vi "capacimetro_adv.vi"() -> ()   [LabVIEW 2019]
uses:
  <vilib>/Analysis/1siggen.llb/Ramp Pattern by Samples.vi
  <vilib>/Instr/_visa.llb/VISA Configure Serial Port (Instr).vi
  <vilib>/Analysis/NI_AALBase.lvlib
  <vilib>/Analysis/NI_AALPro.lvlib
panel:
  out "tau":dbl
  in  "Medie":bool
  out "ADC NL":cluster{dbl[], dbl[]}(graph)
  out "Residui":cluster{dbl[], dbl[]}(graph)
  out "Segnale":cluster{dbl[], "Best Exponential Fit":dbl[]}[](graph)
  out "C[pF]":dbl
  in  "Rs[kohm]":dbl
  out "offset":dbl
  in  "dT":i32
  in  "begin":i32
  in  "length":i32
  in  "stop":bool
  in  "VISA resource name":refnum<visa-resource-name>
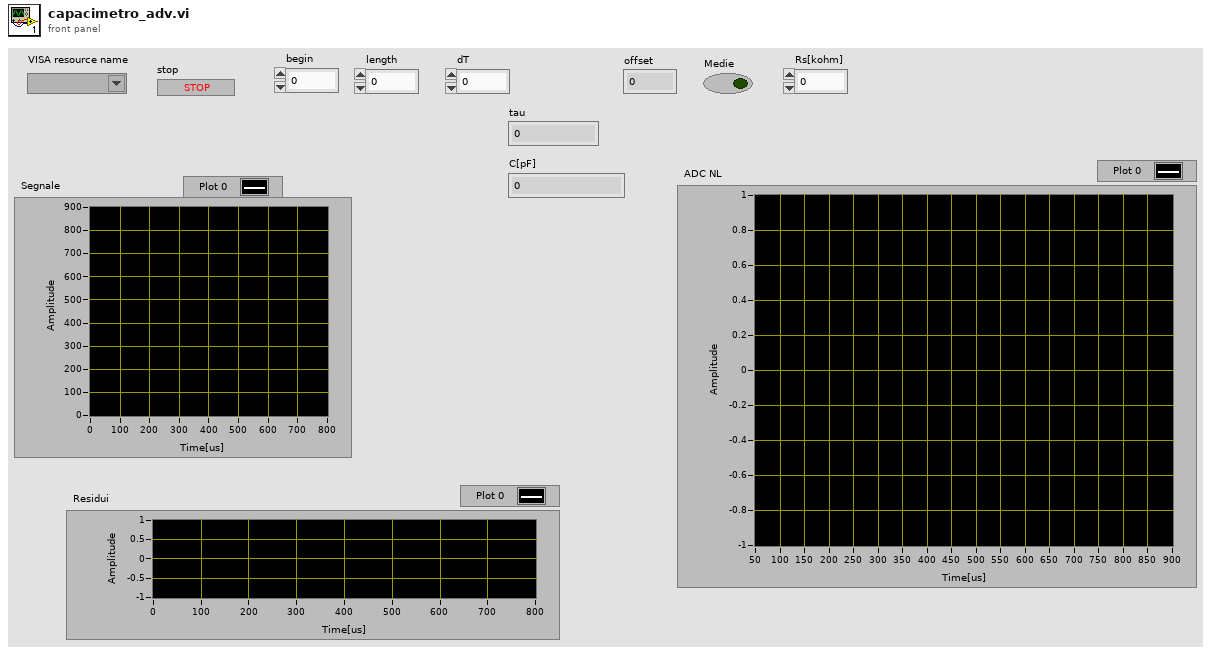
[diagram p1: front panel]
types:
  T1 = cluster{"amp min":dbl, "amp max":dbl, "damping min":dbl, "damping max":dbl, "offset min":dbl, "offset max":dbl}
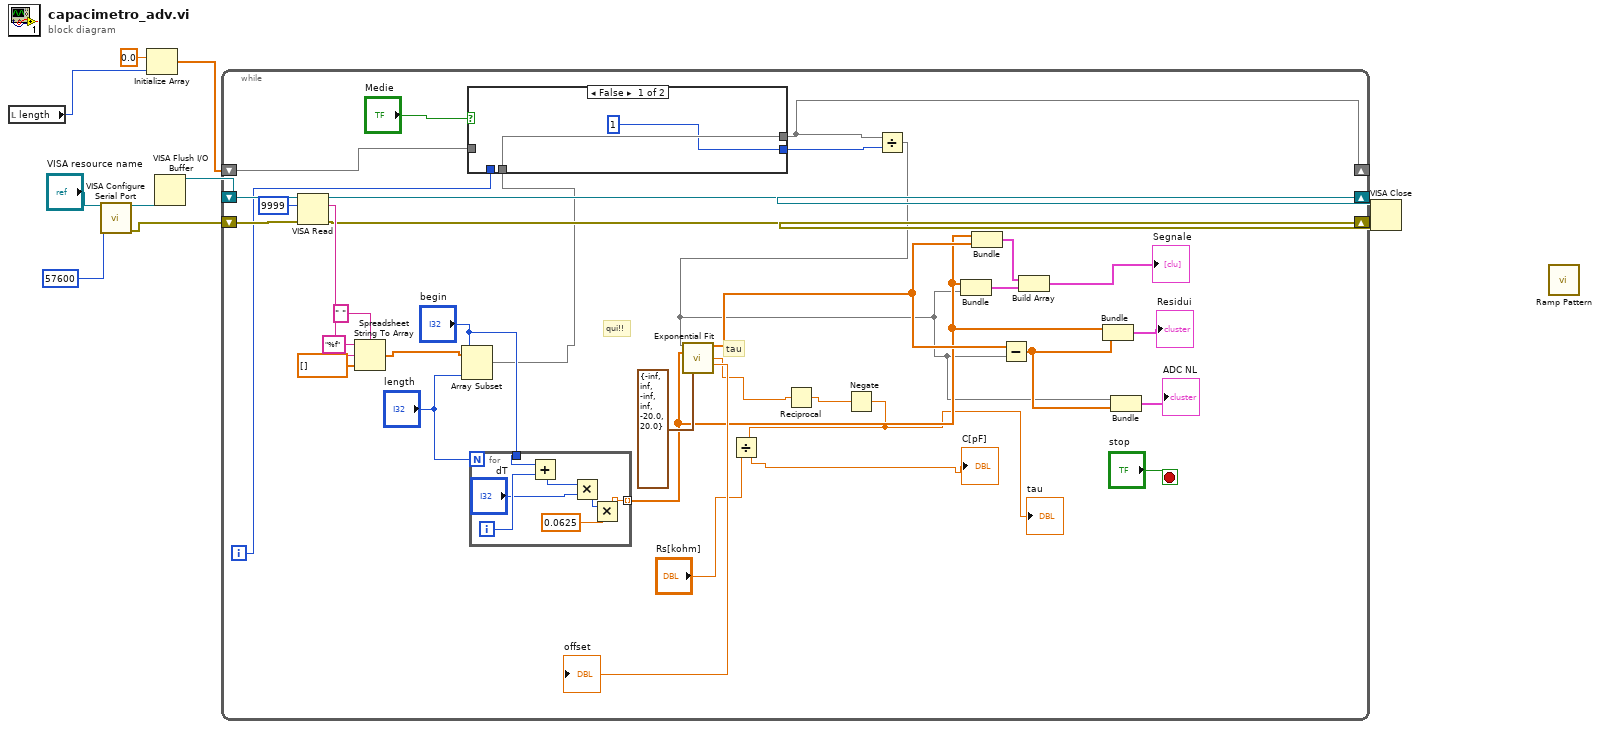
[diagram p0: block diagram]
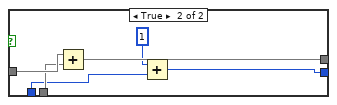
[diagram p2: hidden frame]
diagram:
  n1 = local read "length"() -> (w1:i32)
  n2 = call-poly "VISA Configure Serial Port"("VISA resource name"="VISA resource name", "baud rate (9600)"=u32 57600) -> ("VISA resource name out"=w6:refnum<visa-resource-name>, "error out"=w4:errorcluster)  [unwired: 8 in, 4 out]
  n3 = Initialize Array(0.0 ("element"), w1) -> (w2:dbl[])
  n4 = VISA Flush I/O Buffer(VISA resource name=w6) -> (VISA resource name out=w5:refnum<visa-resource-name>)  [unwired: 2 in, 1 out]
  n5 = while {
    shift-right: [w34] -> w8
    shift-left: w5 -> [w45]
    shift-right: [w33] -> w7
    shift-left: w4 -> [w44]
    shift-right: [w17] -> _
    shift-left: w2 -> [w20]
    i -> [w18]
    stop <- "stop" stop-if-true
    # "tau"
    # "qui!!"
    n6 = VISA Read(VISA resource name=w45, byte count=u32 9999, error in (no error)=w44) -> (VISA resource name out=w34:refnum<visa-resource-name>, read buffer=w41:string, error out=w33:errorcluster)  [unwired: 1 out]
    n7 = Spreadsheet String To Array(delimiter (Tab)=" ", format string="%f", spreadsheet string=w41, array type (2D Dbl)=dbl[] []) -> (array=w37:dbl[])
    n8 = Array Subset(array=w37, index="begin", length="length") -> (w19:dbl[])
    n9 = case shown="False" "Medie" {
      tunnel: w20 -> [_ w53]
      tunnel: w19 -> [w47 w52]
      tunnel: [w47 w51] -> w17
      tunnel: [1 w48] -> w16
      tunnel: w18 -> [_ w50]
      frame False {
      }
      frame True {
        n10 = Add(x=w53, y=w52) -> (x+y=w51:dbl[])
        n11 = Add(x=1, y=w50) -> (x+y=w48:i32)
      }
    }
    n12 = for {
      N: "length" -> [_]
      tunnel: "begin" -> [w59]
      tunnel: [w56] -> w24 mode=indexing
      i -> [w60]
      n13 = Add(x=w59, y=w60) -> (x+y=w58:i32)
      n14 = Multiply(x=w58, y="dT") -> (x*y=w54:i32)
      n15 = Multiply(x=w54, y=0.0625) -> (x*y=w56:dbl)
    }
    n16 = Divide(x=w17, y=w16) -> (x/y=w11:dbl[])
    n17 = call <vilib>:"Exponential Fit.vi"("Y"=w11, "X"=w24, "parameter bounds"=T1 {"amp min"=-inf, "amp max"=inf, "damping min"=-inf, "damping max"=inf, "offset min"=-20.0, "offset max"=20.0}) -> ("Best Exponential Fit"=w26:dbl[], "damping"=w14:dbl, "offset"=→"offset":dbl)  [unwired: 7 in, 3 out]
    n18 = Reciprocal(x=w14) -> (1/x=w13:dbl)
    n19 = Negate(x=w13) -> (-x=w12:dbl)
    "tau" <- w12
    n20 = Divide(x=w12, y="Rs[kohm]") -> (x/y=→"C[pF]":dbl)
    n21 = Bundle(w24, w11) -> (w28:cluster{dbl[], dbl[]})  [unwired: 1 in]
    n22 = Bundle(w24, "Best Exponential Fit"=w26) -> (w29:cluster{dbl[], "Best Exponential Fit":dbl[]})  [unwired: 1 in]
    n23 = Subtract(x=w26, y=w11) -> (x-y=w23:dbl[])
    n24 = Build Array(w29, w28) -> (→"Segnale":cluster{dbl[], "Best Exponential Fit":dbl[]}[])
    n25 = Bundle(w24, w23) -> (→"Residui":cluster{dbl[], dbl[]})  [unwired: 1 in]
    n26 = Bundle(w11, w23) -> (→"ADC NL":cluster{dbl[], dbl[]})  [unwired: 1 in]
  }
  n27 = VISA Close(VISA resource name=w8, error in (no error)=w7) -> ()  [unwired: 1 out]
  n28 = call-poly <vilib>:"Ramp Pattern.vi"() -> ()  [unwired: 10 in, 2 out]
